vi "CRYLoad Virtual Data.vi"(8 "error in":errorcluster) -> (0 "error out":errorcluster)   [LabVIEW 2013]
uses:
  CRYMainGlobal.vi
  CRYMisc vis settings global.vi
panel:
  # "Virtual Data Loading"
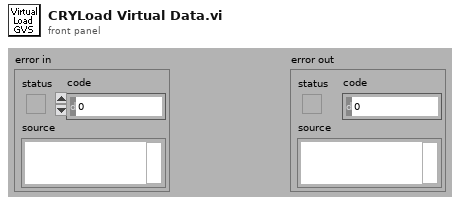
[diagram p1: front panel]
types:
  T1 = enum16{"open", "replace", "create", "open or create", "replace or create", "replace or create with confirmation"}
  T2 = cluster{"Sinal Gen":string, "RTA":string, "Scope-FFT":string, "Voltmeter":string}
  T3 = enum16{"big-endian, network order", "native, host order", "little-endian"}
  T4 = cluster{"gen'r mode":i32, "frequency":u32, "output level":dbl, "wave path":string, "wav play mode":i32, "duration":dbl, "n times":i32, "channel":i32, "wav level":dbl, "EQ":bool, "f knob log":bool, "f knob low":dbl, "f knob high":dbl, "ol knob log":bool, "ol knob low":dbl, "ol knob high":dbl, "Lin Display Prefs":string, "dB Display Prefs":string, "Duration noise":dbl, "Min freq noise":dbl, "Max freq noise":dbl, "Channel String":string, "Play Sine Wave":i32}
  T5 = cluster{"octave":i32, "det time":i32, "det sec":dbl, "lin/exp":i32, "weighting":i32, "channel":i32, "Ave/Max/Min":u16, "continuous":bool, "Applay Correction":bool, "Display":u16, "Channel String":string}
  T6 = typedef "CRYScope-FFT.ctl" = cluster{"window":i32, "n avgs":i32, "lin/exp avg":i32, "pwr/cplx avg":i32, "time (ms)":dbl, "fft lines":i32, "scope/fft mode":i32, "channel":i32, "trig. channel":i32, "Applay Correction":bool, "Time Display":string, "Freq. Weighting":string, "Ave/Max/Min":u16, "Trigger Level":dbl, "Trigger Unit":u16, "Trigger Time Offset":dbl, "Trigger Slope":u16, "Trigger/Free Run":bool, "continuous":bool, "Spectrum Display":string, "Calc FFT":bool, "Y-axis":string, "Signal Type":string}
  T7 = typedef "CRYMultimeter.ctl" = cluster{"Ave/Max/Min":i32, "Level":i32, "Channel":i32, "Signal Type":string, "Weighting":string, "Applay Correction":bool, "lin/exp avg":u16, "rec time (sec)":dbl, "Average Time (Sec)":dbl, "Lin Display Prefs":string, "dB Display Prefs":string, "Time Weighting":u16, "Display":u16}
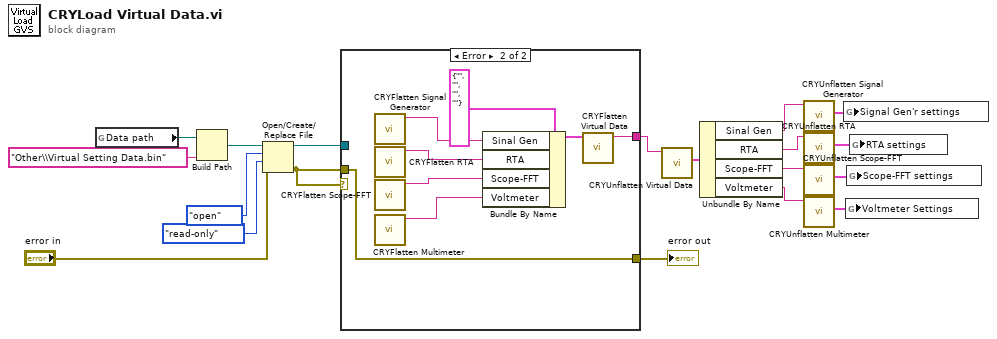
[diagram p0: block diagram]
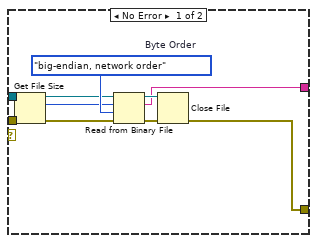
[diagram p2: hidden frame]
diagram:
  n1 = global read "CRYMainGlobal.vi" "Data path"() -> (w1:path)
  n2 = Build Path(base path=w1, name or relative path="Other\\Virtual Setting Data.bin") -> (appended path=w2:path)
  n3 = Open/Create/Replace File(file path (use dialog)=w2, error in="error in", operation (0:open)=T1."open", access (0:read/write)=enum16{"read/write", "read-only", "write-only"}."read-only") -> (refnum out=w15:refnum<file>, error out=w5:errorcluster)  [unwired: 3 out]
  n4 = case shown="Error" w5 {
    tunnel: w5 -> [w26 w36]
    tunnel: [w24 w35] -> w16
    tunnel: w15 -> [w23 _]
    tunnel: [w20 w36] -> w6
    frame No Error {
      w28 = T3."big-endian, network order"  # Byte Order
      n5 = Get File Size(file=w23) -> (refnum out=w22:refnum<file>, size (in bytes)=w21:i64)  [unwired: 1 in, 1 out]
      n6 = Read from Binary File(8:w26, 9:w28, 10:w21, 11:w22) -> (0:w25:errorcluster, 2:w24:string, 3:w27:refnum<file>)  [unwired: 3 out]
      n7 = Close File(refnum=w27, error in=w25) -> (error out=w20:errorcluster)  [unwired: 1 out]
    }
    frame Error {
      n8 = call "CRYFlatten Signal Generator.vi"() -> ("Flat Signal Gen'r settings"=w29:string)  [unwired: 1 in, 10 out]
      n9 = call "CRYFlatten RTA.vi"() -> ("Flat RTA settings"=w30:string)  [unwired: 1 in, 10 out]
      n10 = call "CRYFlatten Scope-FFT.vi"() -> ("Flat Scope-FFT settings"=w31:string)  [unwired: 1 in, 10 out]
      n11 = call "CRYFlatten Multimeter.vi"() -> ("Flat Voltmeter setup"=w32:string)  [unwired: 1 in, 10 out]
      n12 = Bundle By Name(cluster=T2 {"Sinal Gen"="", "RTA"="", "Scope-FFT"="", "Voltmeter"=""} ("Virtual Settings"), "Sinal Gen"=w29, "RTA"=w30, "Scope-FFT"=w31, "Voltmeter"=w32) -> (w33:T2)
      n13 = call "CRYFlatten Virtual Data.vi"("Virtual cluster"=w33) -> ("Flat Virtual Settings"=w35:string)  [unwired: 10 out]
    }
  }
  "error out" <- w6
  n14 = call "CRYUnflatten Virtual Data.vi"("Flatten Virtual"=w16) -> ("Virtual Settings"=w14:T2)  [unwired: 10 out]
  n15 = Unbundle By Name(w14) -> ("Sinal Gen"=w13:string, "RTA"=w12:string, "Scope-FFT"=w10:string, "Voltmeter"=w11:string)
  n16 = call "CRYUnflatten Signal Generator.vi"("Flat Signal Gen'r settings"=w13) -> ("Signal Gen'r settings"=w3:T4)  [unwired: 10 out]
  n17 = call "CRYUnflatten RTA.vi"("Flat RTA setup"=w12) -> ("RTA settings"=w9:T5)  [unwired: 10 out]
  n18 = call "CRYUnflatten Scope-FFT.vi"("Flat Scope-FFT setup"=w10) -> ("Scope-FFT settings"=w8:T6)  [unwired: 10 out]
  n19 = call "CRYUnflatten Multimeter.vi"("Flat Voltmeter setup"=w11) -> ("Voltmeter Settings"=w4:T7)  [unwired: 10 out]
  n20 = global write "CRYMisc vis settings global.vi" "Signal Gen'r settings"(w3) -> ()
  n21 = global write "CRYMisc vis settings global.vi" "Voltmeter Settings"(w4) -> ()
  n22 = global write "CRYMisc vis settings global.vi" "Scope-FFT settings"(w8) -> ()
  n23 = global write "CRYMisc vis settings global.vi" "RTA settings"(w9) -> ()
